vi "14-1.vi"() -> ()   [LabVIEW 2019, in "14.lvlib"]
uses:
  <userlib>/_OpenG.lib/array/array.llb/Remove Duplicates from 1D Array (String)__ogtk.vi
  14.lvlib
panel:
  out "difference":i32
  out "String":string
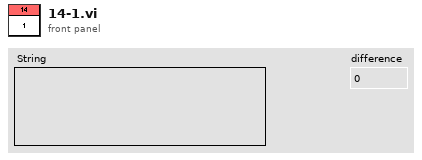
[diagram p1: front panel]
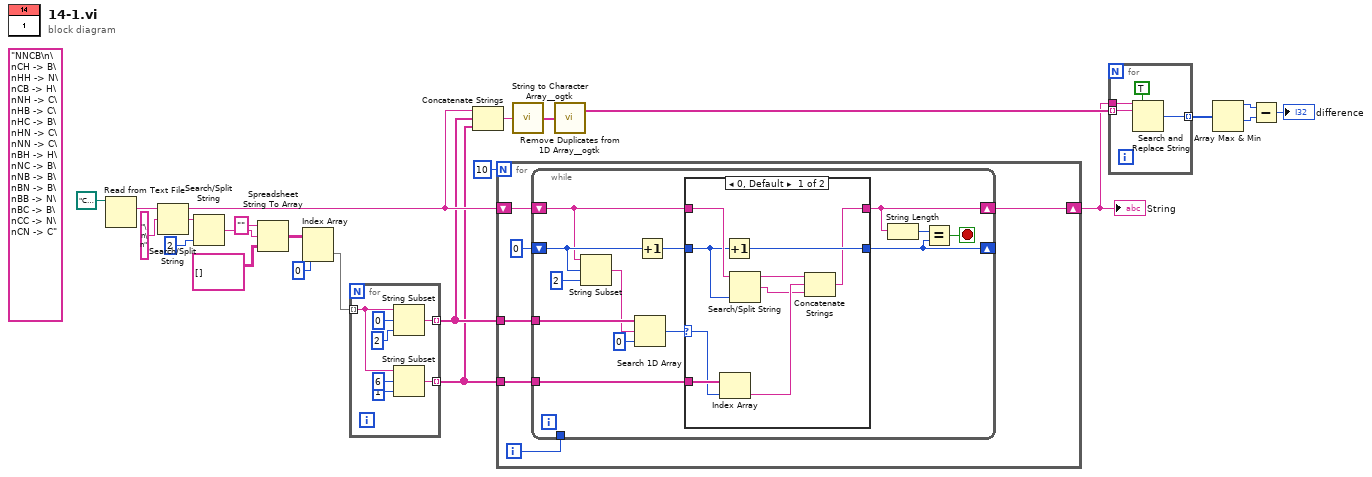
[diagram p0: block diagram]
diagram:
  (unwired) "NNCB\n\nCH -> B\nHH -> N\nCB -> H\nNH -> C\nHB -> C\nHC -> B\nHN -> C\nNN -> C\nBH -> H\nNC -> B\nNB -> B\nBN -> B\nBB -> N\nBC -> B\nCC -> N\nCN -> C"
  n1 = Read from Text File(file (use dialog)=path "C:/Users/craig.walker/Documents/GitHub/lv2019-Advent-of-Code-2021/14/input.txt") -> (text=w1:string)  [unwired: 3 in, 3 out]
  n2 = Search/Split String(string=w1, search string/char (-)="\n\n") -> (substring before match=w13:string, match + rest of string=w21:string)  [unwired: 1 in, 1 out]
  n3 = Search/Split String(string=w21, offset (0)=2) -> (match + rest of string=w19:string)  [unwired: 1 in, 2 out]
  n4 = Spreadsheet String To Array(format string="", spreadsheet string=w19, array type (2D Dbl)=string[][] [] ("search string/char (-)")) -> (array=w16:string[][])  [unwired: 1 in]
  n5 = Index Array(array=w16, index (col)=0 ("disabled index (col)")) -> (element=w17:string[])  [unwired: 1 in]
  n6 = for {
    tunnel: w17 -> [w28] mode=indexing
    tunnel: [w25] -> w12 mode=indexing
    tunnel: [w24] -> w11 mode=indexing
    n7 = String Subset(string=w28, offset (0)=0, length (rest)=2 ("length (rest)")) -> (substring=w25:string)
    n8 = String Subset(string=w28, offset (0)=6, length (rest)=1 ("length (rest)")) -> (substring=w24:string)
  }
  n9 = Concatenate Strings(w13, w12, w11) -> (w10:string)
  n10 = for {
    N: 10 -> [_]
    shift-right: [w32] -> w2
    shift-left: w13 -> [w36]
    tunnel: w12 -> [w34]
    tunnel: w11 -> [w33]
    i -> [w31]
    n11 = while {
      shift-right: [w39] -> _
      shift-left: u64 0 ("offset (0)") -> [w45]
      tunnel: w34 -> [w48]
      shift-right: [w41] -> w32
      shift-left: w36 -> [w44]
      tunnel: w33 -> [w42]
      tunnel: w31 -> [_]
      stop <- w38 stop-if-true
      n12 = String Subset(string=w44, offset (0)=w45, length (rest)=2 ("length (rest)")) -> (substring=w47:string)
      n13 = Search 1D Array(1D array=w48, element=w47, start index (0)=u64 0) -> (index of element=w46:i32)
      n14 = Increment(x=w45) -> (x+1=w43:u64)
      n15 = case shown="0, Default" w46 {
        selector: w46 -> [w57 _]
        tunnel: w44 -> [w55 w60]
        tunnel: [w51 w60] -> w41
        tunnel: w43 -> [w54 w59]
        tunnel: [w56 w59] -> w39
        tunnel: w42 -> [w58 _]
        frame 0, Default {
          n16 = Index Array(array=w58, index=w57) -> (element=w53:string)
          n17 = Increment(x=w54) -> (x+1=w56:u64)
          n18 = Search/Split String(string=w55, offset (0)=w54) -> (substring before match=w52:string, match + rest of string=w50:string)  [unwired: 1 in, 1 out]
          n19 = Concatenate Strings(w52, w53, w50) -> (w51:string)
        }
        frame -1 {
        }
      }
      n20 = String Length(string=w41) -> (length=w40:i32)
      n21 = Equal?(x=w40, y=w39) -> (x = y?=w38:bool)
    }
  }
  "String" <- w2
  n22 = call <userlib>:"String to Character Array__ogtk.vi"("Input String"=w10) -> ("Character Array"=w9:string[])
  n23 = call-poly <userlib>:"Remove Duplicates from 1D Array__ogtk.vi"("Input Array"=w9) -> ("Output Array"=w8:string[])  [unwired: 1 out]
  n24 = for {
    tunnel: w2 -> [w64]
    tunnel: w8 -> [w63] mode=indexing
    tunnel: [w62] -> w7 mode=indexing
    n25 = Search and Replace String(replace all?=TRUE ("replace all? (F)"), input string=w64, search string=w63) -> (number of replacements=w62:i32)  [unwired: 5 in, 3 out]
  }
  n26 = Array Max & Min(array=w7) -> (max value=w6:i32, min value=w5:i32)  [unwired: 2 out]
  n27 = Subtract(x=w6, y=w5) -> (x-y=→"difference":i32)
